vi "Launch Wait on Listener.vi"(9 "Endpoint":refnum<class "Endpoint.lvclass">, 10 "Listener Notifier":T1, 11 "Listener":refnum<k5>) -> ()   [LabVIEW 2020, in "Stream-TCP.lvlib" / "TCP Client.lvclass"]
uses:
  TCP Client.lvclass
  Listener Notifier.ctl
  Listener Status.ctl
  lv-stream/stream/Endpoint/Endpoint.lvclass
  lv-stream/stream/Connection State.ctl
  C:/dev/LabVIEW/lv-stream/stream/Endpoint/Endpoint.lvclass
  C:/dev/LabVIEW/lv-stream/stream/Connection/Connection.lvclass
  Stream-TCP.lvlib
  lv-stream/stream/Connection/Connection.lvclass
  lv-stream/stream/Stream.lvlib
panel:
  out "URI String":string
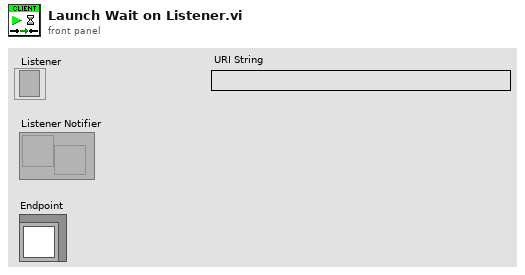
[diagram p1: front panel]
types:
  T1 = typedef "Stream-TCP.lvlib/Listener Notifier.ctl" = refnum<notifier>
  T2 = typedef "Stream-TCP.lvlib/Listener Status.ctl" = enum16{"Successful", "Unsuccessful"}
  T3 = typedef "Stream.lvlib/Connection State.ctl" = enum16{"Connected", "Disconnected"}
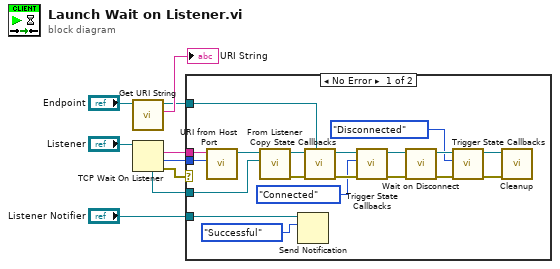
[diagram p0: block diagram]
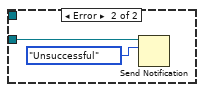
[diagram p2: hidden frame]
diagram:
  n1 = call "Get URI String.vi"("Endpoint in"="Endpoint") -> ("URI String"=→"URI String":string, "Endpoint out"=w1:refnum<class "Endpoint.lvclass">)  [unwired: 8 in, 1 out]
  n2 = TCP Wait On Listener(11:"Listener") -> (0:w6:errorcluster, 1:w3:u16, 2:w4:string, 4:w5:refnum<k5>)  [unwired: 3 in, 1 out]
  n3 = case shown="No Error" w6 {
    tunnel: w5 -> [w25 _]
    tunnel: w4 -> [w28 _]
    tunnel: w3 -> [w27 _]
    tunnel: "Listener Notifier" -> [w13 w30]
    tunnel: w1 -> [w23 _]
    frame No Error {
      n4 = call "URI from Host Port.vi"("Port"=w27, "Host"=w28) -> ("URI"=w26:refnum<class "URI.lvclass">)  [unwired: 9 in]
      n5 = call "From Listener.vi"("TCP Connection"=w25, "URI"=w26) -> ("error out"=w22:errorcluster, "TCP Client"=w24:refnum<class "TCP Client.lvclass">)  [unwired: 8 in]
      n6 = Send Notification(notification=Listener_Status."Successful", notifier=w13) -> ()  [unwired: 1 in, 2 out]
      n7 = call "Copy State Callbacks.vi"("From"=w23, "error in (no error)"=w22, "Endpoint in"=w24) -> ("error out"=w20:errorcluster, "Endpoint out"=w21:refnum<class "TCP Client.lvclass">)  [unwired: 7 in]
      n8 = call "Trigger State Callbacks.vi"("error in (no error)"=w20, "State"=Connection_State."Connected", "Connection in"=w21) -> ("error out"=w18:errorcluster, "Connection out"=w17:refnum<class "TCP Client.lvclass">)  [unwired: 7 in]
      n9 = call "Wait on Disconnect.vi"("error in (no error)"=w18, "TCP Client in"=w17) -> ("error out"=w16:errorcluster, "TCP Client out"=w15:refnum<class "TCP Client.lvclass">)  [unwired: 8 in]
      n10 = call "Trigger State Callbacks.vi"("error in (no error)"=w16, "State"=Connection_State."Disconnected", "Connection in"=w15) -> ("error out"=w11:errorcluster, "Connection out"=w10:refnum<class "TCP Client.lvclass">)  [unwired: 7 in]
      n11 = call-dynamic "Cleanup.vi"("error in (no error)"=w11, "TCP Client in"=w10) -> ()  [unwired: 9 in, 1 out]
    }
    frame Error {
      n12 = Send Notification(notification=Listener_Status."Unsuccessful", notifier=w30) -> ()  [unwired: 1 in, 2 out]
    }
  }
